vi "Result All Modes.vi"() -> ()   [LabVIEW 2025]
uses:
  <instrlib>/Chroma 19052/Chroma 19052.lvlib
panel:
  out "Results":string
  out "VISA resource name out":refnum<visa-resource-name>
  in  "VISA resource name":refnum<visa-resource-name>
  out "error out":errorcluster
  in  "error in (no error)":errorcluster
  # "Result All Mode?"
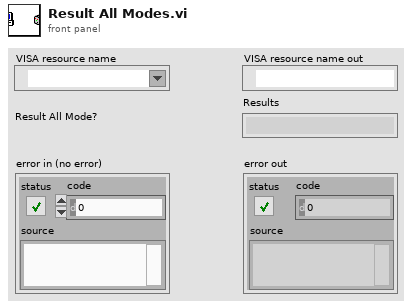
[diagram p1: front panel]
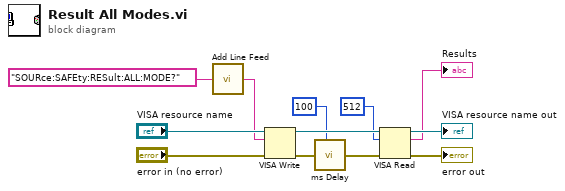
[diagram p0: block diagram]
diagram:
  n1 = call <instrlib>:"Add Line Feed.vi"("Command string"="SOURce:SAFEty:RESult:ALL:MODE?") -> ("Concatenated string"=w9:string)  [unwired: 4 in]
  n2 = VISA Write(VISA resource name="VISA resource name", write buffer=w9, error in (no error)="error in (no error)") -> (VISA resource name out=w11:refnum<visa-resource-name>, error out=w3:errorcluster)  [unwired: 1 out]
  n3 = call <instrlib>:"ms Delay.vi"("miliseconds to wait"=u32 100, "error in (no error)"=w3) -> ("error out"=w2:errorcluster)  [unwired: 6 in, 1 out]
  n4 = VISA Read(VISA resource name=w11, byte count=u32 512, error in (no error)=w2) -> (VISA resource name out=→"VISA resource name out":refnum<visa-resource-name>, read buffer=→"Results":string, error out=→"error out":errorcluster)  [unwired: 1 out]
